vi "HTS221 Example.vi"() -> ()   [LabVIEW 2020]
uses:
  HTS221/HTS221 Data Rates.ctl
  <vilib>/MakerHub/LINX/Public/Utilities/Open Local.vi
  LINX I2C/LINX I2C.lvclass
  <vilib>/MakerHub/LINX/LMH-LINX.lvlib
  HTS221/HTS221.lvclass
panel:
  out "Relative Humidity (%)":dbl
  out "Temperature (degC)":dbl
  in  "stop":bool
  out "Waveform Chart":dbl[][](graph)
  out "Error Out":errorcluster
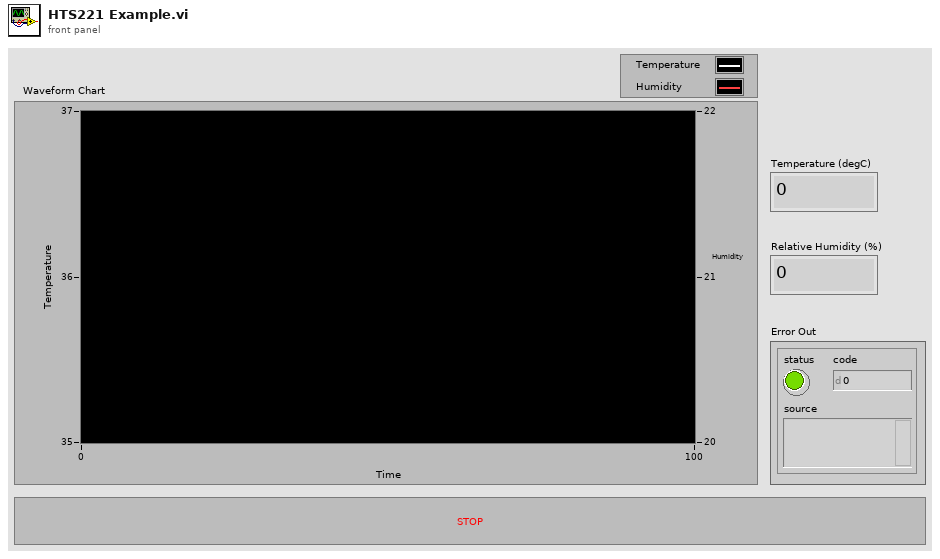
[diagram p1: front panel]
types:
  T1 = typedef "HTS221.lvclass/HTS221 Data Rates.ctl" = enum16{"One-Shot", "1Hz", "7Hz", "12.5Hz"}
  T2 = typedef "LMH-LINX.lvlib/LINX Ref.ctl" = cluster{"IO":T3, "Interface":T4, "LINX Device Config":T5}
  T3 = typedef "LMH-LINX.lvlib/Platform.ctl" = enum16{"Remote", "Local"}
  T4 = typedef "LMH-LINX.lvlib/Interface.ctl" = enum16{"Serial", "TCP"}
  T5 = typedef "LMH-LINX.lvlib/Device.lvlib/LINX Device Config.ctl" = cluster{"Interface":T4, "COM Port":refnum<visa-resource-name>, "TCP Configuration":T6, "Device Family":u8, "Device ID":u8, "Device Name":string, "TCP Ref":refnum<k5>, "Channels":T7}
  T6 = typedef "LMH-LINX.lvlib/Device.lvlib/TCP Config.ctl" = cluster{"IP Address":string, "Port":u16}
  T7 = typedef "LMH-LINX.lvlib/Channels.ctl" = cluster{"DI":u8[], "DO":u8[], "AI":u8[], "AO":u8[], "PWM":u8[], "QE":u8[], "UART":u8[], "I2C 2":u8[], "SPI":u8[], "CAN":u8[], "Servo":u8[], "AI Ref (V)":dbl, "AI Resolution (Bits)":u8, "AO Ref (V)":dbl, "AO Resolution (Bits)":u8}
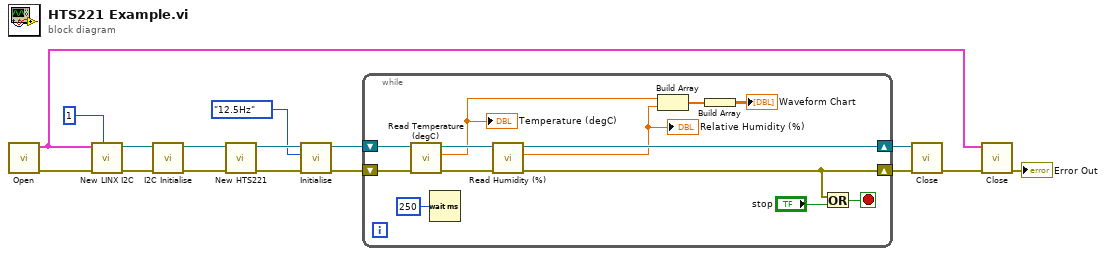
[diagram p0: block diagram]
diagram:
  n1 = call-poly <vilib>:"Open.vi"() -> ("Error Out"=w15:errorcluster, "LINX Resource"=w11:T2)  [unwired: 9 in, 1 out]
  n2 = call "New LINX I2C.vi"("LINX I2C Channel"=u8 1 ("I2C Channel"), "error in (no error)"=w15, "LINX Resource"=w11) -> ("error out"=w13:errorcluster, "LINX I2C out"=w12:refnum<class "LINX I2C.lvclass">)  [unwired: 7 in]
  n3 = call-dynamic "I2C Initialise.vi"("error in (no error)"=w13, "LINX I2C in"=w12) -> ("error out"=w8:errorcluster, "LINX I2C out"=w7:refnum<class "LINX I2C.lvclass">)  [unwired: 8 in]
  n4 = call "New HTS221.vi"("error in (no error)"=w8, "I2C in"=w7) -> ("error out"=w6:errorcluster, "HTS221 out"=w5:refnum<class "HTS221.lvclass">)  [unwired: 8 in]
  n5 = call "Initialise.vi"("error in (no error)"=w6, "Data Rate (12.5Hz)"=HTS221_Data_Rates."12.5Hz" ("Data Rate (1Hz)"), "HTS221 in"=w5) -> ("error out"=w10:errorcluster, "HTS221 out"=w9:refnum<class "HTS221.lvclass">)  [unwired: 7 in]
  n6 = while {
    shift-right: [w20] -> w3
    shift-left: w10 -> [w24]
    shift-right: [w21] -> w4
    shift-left: w9 -> [w25]
    stop <- w28 stop-if-true
    n7 = call "Read Temperature (degC).vi"("error in (no error)"=w24, "HTS221 in"=w25) -> ("error out"=w22:errorcluster, "Temperature (degC)"=w18:dbl, "HTS221 out"=w23:refnum<class "HTS221.lvclass">)  [unwired: 7 in]
    "Temperature (degC)" <- w18
    n8 = Wait (ms)(milliseconds to wait=u32 250) -> ()  [unwired: 1 out]
    n9 = call "Read Humidity (%).vi"("error in (no error)"=w22, "HTS221 in"=w23) -> ("error out"=w20:errorcluster, "Relative Humidity (%)"=w19:dbl, "HTS221 out"=w21:refnum<class "HTS221.lvclass">)  [unwired: 7 in]
    "Relative Humidity (%)" <- w19
    n10 = Build Array(w18, w19) -> (w17:dbl[])
    n11 = Build Array(w17) -> (→"Waveform Chart":dbl[][])
    n12 = Or(x=w20, y="stop") -> (x .or. y?=w28:bool)
  }
  n13 = call <vilib>:"Close.vi"("error in (no error)"=w3, "HTS221 in"=w4) -> ("error out"=w2:errorcluster)  [unwired: 8 in, 1 out]
  n14 = call <vilib>:"Close.vi"("Error In"=w2, "LINX Resource"=w11) -> ("Error Out"=→"Error Out":errorcluster)  [unwired: 9 in]
